vi "recording-audio-queued].vi"() -> ()   [LabVIEW 2021]
uses:
  <vilib>/sound2/lvsound2.llb/Sound Data Format.ctl
  <vilib>/sound2/lvsound2.llb/Sampling Mode.ctl
  <vilib>/sound2/lvsound2.llb/Sound File Write Open.vi
  <vilib>/sound2/lvsound2.llb/Sound File Write (DBL).vi
  <vilib>/sound2/lvsound2.llb/Sound Input Read (DBL).vi
panel:
  out "Error Loop 2":bool
  out "Error Loop 1":bool
  out "Waveform Graph":waveform(dbl)[](graph)
  in  "Sound Format":T1={"sample rate (S/s)"=22050.0, "number of channels"=2, "bits per sample"=16}
  in  "stop":bool
  in  "Device ID":u32 format="%.0x"
  in  "Number of Samples/ch":i32=10000
  out "Recorded signal without transisent":dynamicdata(graph) caption="Section"
  in  "Discard Transisent":i32 caption="Begin Sample"
  out "Recorded Signal":dynamicdata(graph) caption="Data"
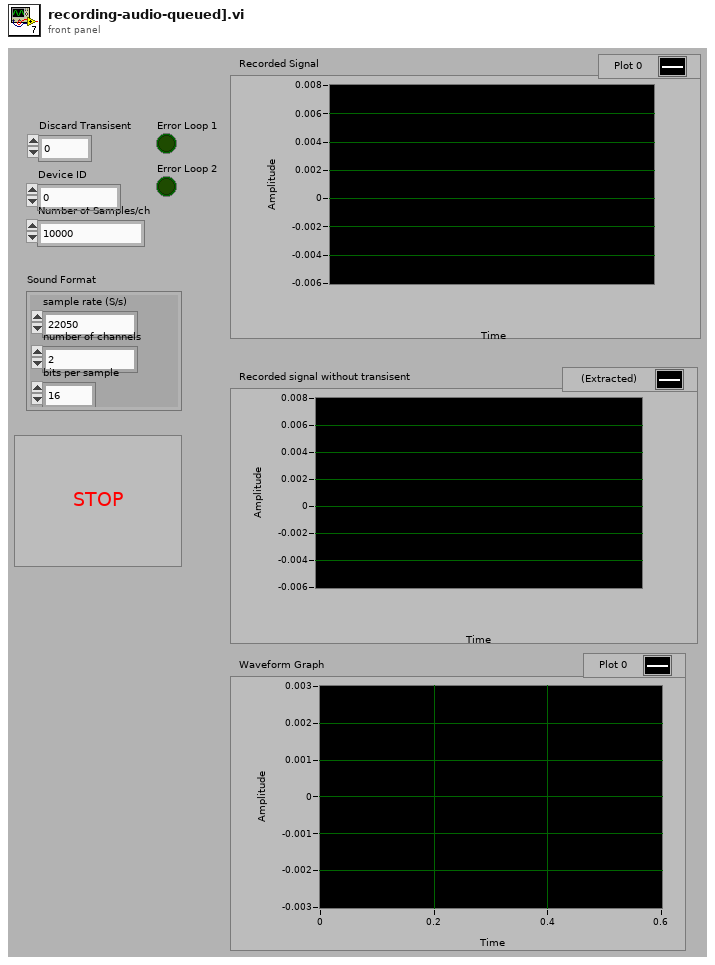
[diagram p1: front panel]
types:
  T1 = typedef "Sound Data Format.ctl" = cluster{"sample rate (S/s)":dbl, "number of channels":i32, "bits per sample":i32}
  T2 = typedef "Sampling Mode.ctl" = i32
  T3 = typedef "Sound File Refnum.ctl" = refnum<file>
  T4 = typedef "Sound Input Task ID.ctl" = u32
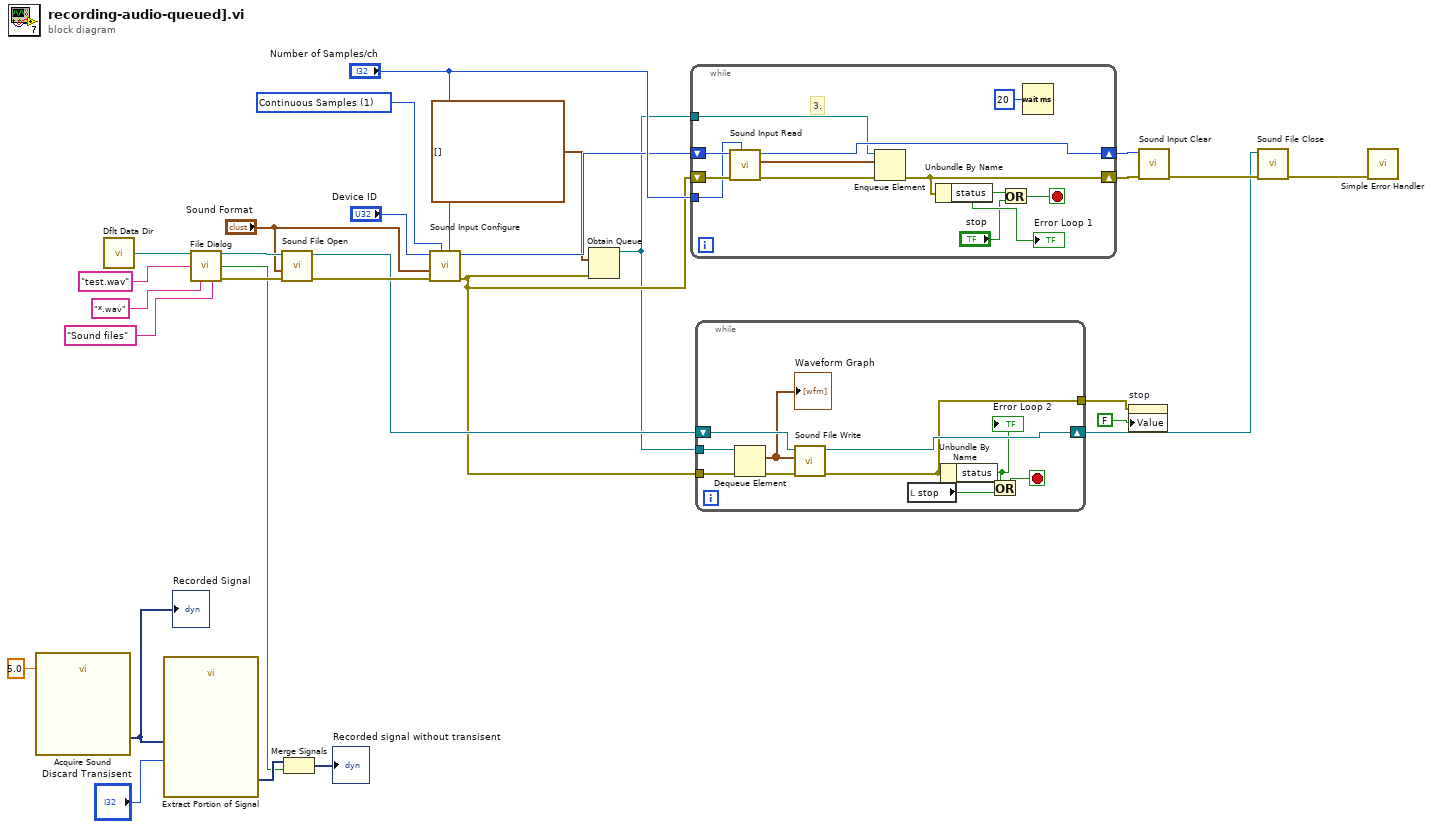
[diagram p0: block diagram]
diagram:
  w16 = T2 1 items=["Finite Samples", "Continuous Samples"] ("sample mode")
  n1 = call "Acquire Sound"("Duration (s)"=5.0) -> ("Data"=w27:dynamicdata)  [unwired: 5 in, 13 out]
  "Recorded Signal" <- w27
  n2 = call <vilib>:"Dflt Data Dir.vi"() -> ("App:Default Data Directory"=w21:path)
  n3 = call "Extract Portion of Signal"("Begin Sample"="Discard Transisent", "Signals"=w27) -> ("Section"=w28:dynamicdata)  [unwired: 1 in, 8 out]
  n4 = call "File Dialog"("start path"=w21, "default name"="test.wav", "pattern (all files)"="*.wav" ("DNL_pattern"), "pattern label"="Sound files") -> ("selected path"=w24:path, "exists"=w9:bool, "error out"=w25:errorcluster)  [unwired: 3 in, 6 out]
  n5 = call-poly <vilib>:"Sound File Open.vi"("error in (no error)"=w25, "sound format"="Sound Format", "path"=w24) -> ("error out"=w18:errorcluster, "sound file refnum"=w7:T3)  [unwired: 7 out]
  n6 = Merge Signals(w28, w9) -> (→"Recorded signal without transisent":dynamicdata)
  n7 = call <vilib>:"Sound Input Configure.vi"("number of samples/ch"="Number of Samples/ch", "sample mode"=w16, "error in (no error)"=w18, "sound format"="Sound Format", "device ID"="Device ID") -> ("error out"=w6:errorcluster, "task ID"=w12:T4)  [unwired: 1 in, 4 out]
  n8 = Obtain Queue(element data type=waveform(dbl)[] [] ("data"), error in (no error)=w6) -> (queue out=w4:refnum<queue>)  [unwired: 2 in, 3 out]
  n9 = while {
    tunnel: "Number of Samples/ch" -> [w38]
    shift-right: [w39] -> w13
    shift-left: w12 -> [w40]
    shift-right: [w31] -> w14
    shift-left: w6 -> [w41]
    tunnel: w4 -> [w32]
    stop <- w35 stop-if-true
    # "3."
    n10 = call-poly <vilib>:"Sound Input Read.vi"("number of samples/ch"=w38, "error in (no error)"=w41, "task ID"=w40) -> ("error out"=w34:errorcluster, "data"=w33:waveform(dbl)[], "task ID out"=w39:T4)  [unwired: 1 in, 5 out]
    n11 = Enqueue Element(queue=w32, element=w33, error in (no error)=w34) -> (error out=w31:errorcluster)  [unwired: 3 out]
    n12 = Unbundle By Name(w31) -> ("status"=w37:bool)
    "Error Loop 1" <- w37
    n13 = Or(x=w37, y="stop") -> (x .or. y?=w35:bool)
    n14 = Wait (ms)(milliseconds to wait=u32 20) -> ()  [unwired: 1 out]
  }
  n15 = while {
    tunnel: w6 -> [w49]
    tunnel: w4 -> [w50]
    shift-right: [w47] -> w3
    shift-left: w7 -> [w51]
    tunnel: [w42] -> w2
    stop <- w44 stop-if-true
    n16 = Dequeue Element(queue=w50, error in (no error)=w49) -> (element=w46:waveform(dbl)[], error out=w48:errorcluster)  [unwired: 3 out]
    "Waveform Graph" <- w46
    n17 = call-poly <vilib>:"Sound File Write.vi"("error in (no error)"=w48, "data"=w46, "sound file refnum"=w51) -> ("error out"=w42:errorcluster, "sound file refnum out"=w47:T3)  [unwired: 7 out]
    n18 = local read "stop"() -> (w45:bool)
    n19 = Unbundle By Name(w42) -> ("status"=w43:bool)
    "Error Loop 2" <- w43
    n20 = Or(x=w43, y=w45) -> (x .or. y?=w44:bool)
  }
  n21 = property on="stop" class="Bool (strict)"(error in=w2, "Value"=FALSE ("stop")) -> ()  [unwired: 1 in, 2 out]
  n22 = call <vilib>:"Sound Input Clear.vi"("error in (no error)"=w14, "task ID"=w13) -> ("error out"=w17:errorcluster)  [unwired: 9 out]
  n23 = call <vilib>:"Sound File Close.vi"("error in (no error)"=w17, "sound file refnum"=w3) -> ("error out"=w19:errorcluster)  [unwired: 9 out]
  n24 = call <vilib>:"Simple Error Handler.vi"("error in (no error)"=w19) -> ()  [unwired: 1 in, 8 out]
